vi "Write Stream Mode Algorithm.vi"(10 "Stream Mode Algorithm":T1, 11 "SwitchToStreamMode in":refnum<class "SwitchToStreamMode.lvclass">) -> (3 "SwitchToStreamMode out":refnum<class "SwitchToStreamMode.lvclass">)   [LabVIEW 2013, in "SwitchToStreamMode.lvclass"]
uses:
  SwitchToStreamMode.lvclass
  Configuration/Stream Mode Algorithm.ctl
  SwitchToStreamMode.lvclass/SwitchToStreamMode.ctl
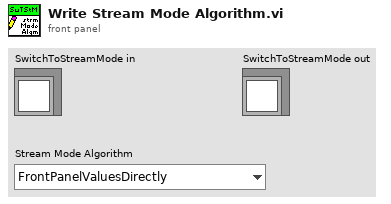
[diagram p1: front panel]
types:
  T1 = typedef "Stream Mode Algorithm.ctl" = enum16{"FrontPanelValuesDirectly"}
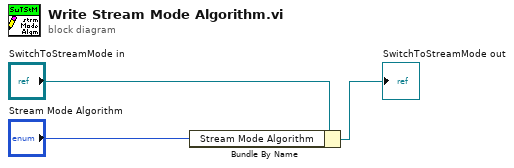
[diagram p0: block diagram]
diagram:
  n1 = Bundle By Name(cluster="SwitchToStreamMode in", "Stream Mode Algorithm"="Stream Mode Algorithm") -> (→"SwitchToStreamMode out":refnum<class "SwitchToStreamMode.lvclass">)
